vi "2.4.vi"() -> ()   [LabVIEW 2020]
panel:
  out "x*y":string
  out "x/y":string
  out "x-y":string
  out "x+y":string
  in  "y":dbl
  in  "x":dbl
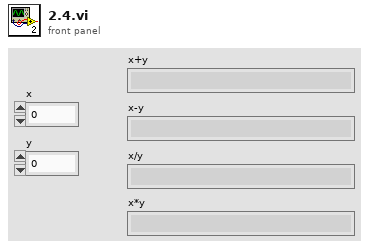
[diagram p1: front panel]
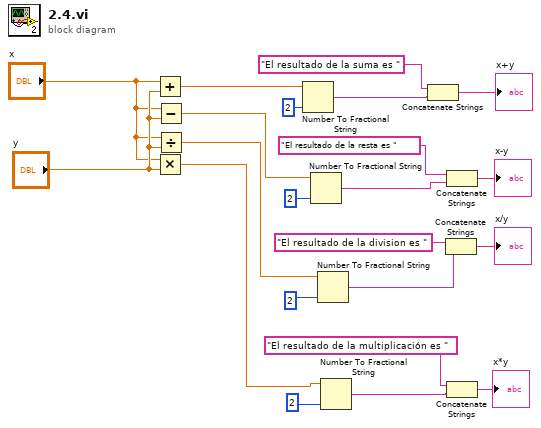
[diagram p0: block diagram]
diagram:
  n1 = Add(x="x", y="y") -> (x+y=w4:dbl)
  n2 = Multiply(x="x", y="y") -> (x*y=w8:dbl)
  n3 = Subtract(x="x", y="y") -> (x-y=w7:dbl)
  n4 = Divide(x="x", y="y") -> (x/y=w11:dbl)
  n5 = Number To Fractional String(number=w4, precision (6)=i16 2 ("width (-)")) -> (F-format string=w5:string)  [unwired: 2 in]
  n6 = Number To Fractional String(number=w7, precision (6)=i16 2 ("width (-)")) -> (F-format string=w6:string)  [unwired: 2 in]
  n7 = Number To Fractional String(number=w11, precision (6)=i16 2 ("width (-)")) -> (F-format string=w12:string)  [unwired: 2 in]
  n8 = Number To Fractional String(number=w8, precision (6)=i16 2 ("width (-)")) -> (F-format string=w10:string)  [unwired: 2 in]
  n9 = Concatenate Strings("El resultado de la suma es ", w5) -> (→"x+y":string)
  n10 = Concatenate Strings("El resultado de la division es ", w12) -> (→"x/y":string)
  n11 = Concatenate Strings("El resultado de la resta es ", w6) -> (→"x-y":string)
  n12 = Concatenate Strings("El resultado de la multiplicación es ", w10) -> (→"x*y":string)
